vi "constants.vi"(8 "error in (no error)":errorcluster, 11 "Small?":bool) -> (0 "error out":errorcluster, 1 "batch updater file path":path, 3 "DB connection File Path":path, 4 "file path for Processed Signal .hdf5 files":path, 5 "Testing":bool=TRUE, 6 "Private Folder file path":path)   [LabVIEW 2013]
doc: "Detects if the computer is on a production computer or a test computer and ouputs paths to various useful locations based on whether or not it is testing."
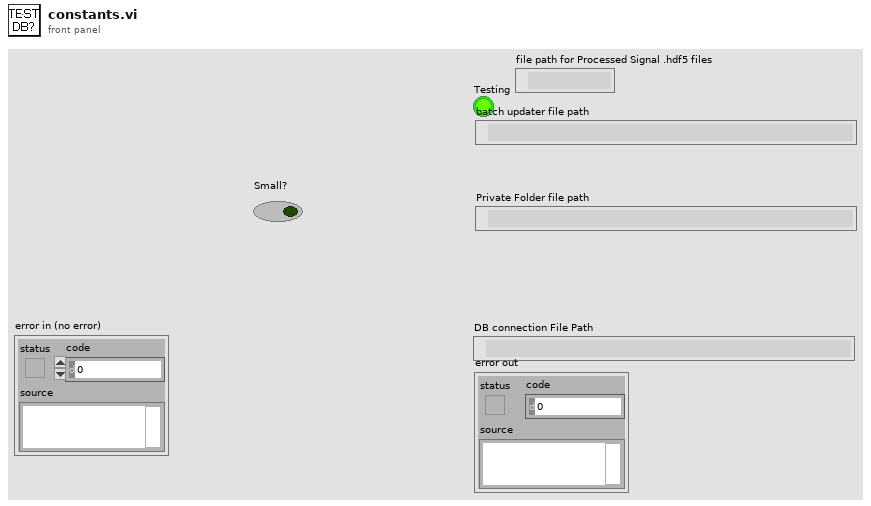
[diagram p1: front panel]
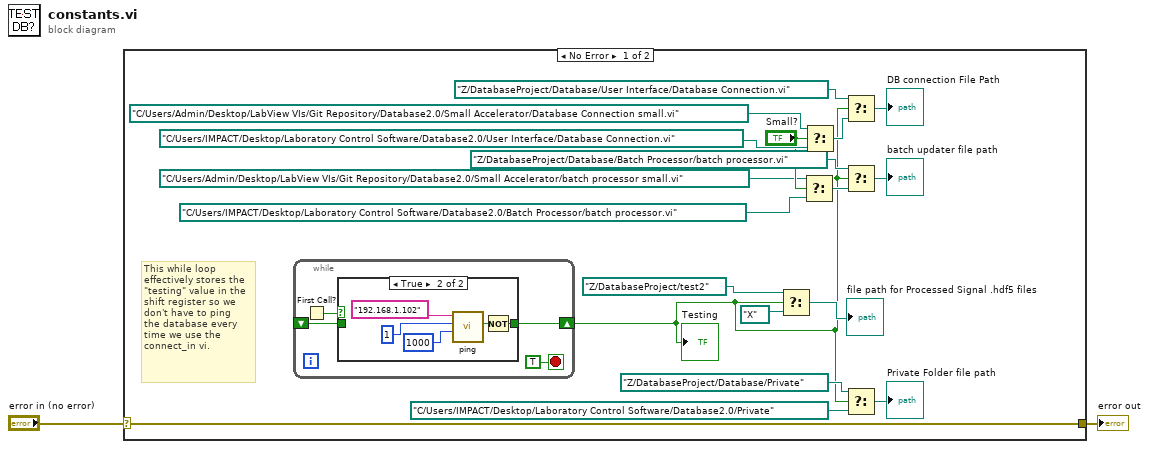
[diagram p0: block diagram]
diagram:
  n1 = case shown="No Error" "error in (no error)" {
    selector: "error in (no error)" -> [w19 w32]
    tunnel: [w19 w32] -> w2
    frame No Error {
      # "This while loop\neffectively stores the\n\"testing\" value in the\nshift register so we\ndon't have to ping\nthe database every\ntime we use the\nconnect_in vi."
      n2 = while {
        shift-right: [w25] -> w3
        shift-left: _ -> [w22]
        stop <- TRUE stop-if-true
        n3 = First Call?() -> (First Call?: T/F=w24:bool)
        n4 = case shown="True" w24 {
          tunnel: [w26 w27] -> w25
          tunnel: w22 -> [w26 _]
          frame False {
          }
          frame True {
            n5 = call "ping.vi"("timeout (ms)"=1000, "count"=1, "host"="192.168.1.102") -> ("found?"=w28:bool)  [unwired: 6 in, 2 out]
            n6 = Not(x=w28) -> (.not. x?=w27:bool)
          }
        }
      }
      "Testing" <- w3
      n7 = Select(t=path "Z:/DatabaseProject/test2", s=w3, f=path "X:/") -> (s? t:f=→"file path for Processed Signal .hdf5 files":path)
      n8 = Select(t=path "C:/Users/Admin/Desktop/LabView VIs/Git Repository/Database2.0/Small Accelerator/batch processor small.vi" ("vi path"), s="Small?", f=path "C:/Users/IMPACT/Desktop/Laboratory Control Software/Database2.0/Batch Processor/batch processor.vi" ("vi path")) -> (s? t:f=w6:path)
      n9 = Select(t=path "C:/Users/Admin/Desktop/LabView VIs/Git Repository/Database2.0/Small Accelerator/Database Connection small.vi" ("vi path"), s="Small?", f=path "C:/Users/IMPACT/Desktop/Laboratory Control Software/Database2.0/User Interface/Database Connection.vi" ("vi path")) -> (s? t:f=w8:path)
      n10 = Select(t=path "Z:/DatabaseProject/Database/User Interface/Database Connection.vi", s=w3, f=w8) -> (s? t:f=→"DB connection File Path":path)
      n11 = Select(t=path "Z:/DatabaseProject/Database/Batch Processor/batch processor.vi", s=w3, f=w6) -> (s? t:f=→"batch updater file path":path)
      n12 = Select(t=path "Z:/DatabaseProject/Database/Private", s=w3, f=path "C:/Users/IMPACT/Desktop/Laboratory Control Software/Database2.0/Private" ("vi path")) -> (s? t:f=→"Private Folder file path":path)
    }
    frame Error {
    }
  }
  "error out" <- w2
